vi "AnalogIO.vi"(0 "a_hDevice":i32) -> ()   [LabVIEW 2016]
panel:
  in  "SetAnalogOut":bool
  in  "GetAnalogIn":bool
  in  "GetOnboardAI":bool
  out "AI0":dbl format="%3.2f"
  out "AI7":dbl format="%.2f"
  out "AI6":dbl format="%.2f"
  out "AI3":dbl format="%.2f"
  out "AI2":dbl format="%.2f"
  out "AI1":dbl format="%.2f"
  out "AI4":dbl format="%.2f"
  out "AI5":dbl format="%.2f"
  in  "AO2":dbl format="%.2f"
  in  "AO1":dbl format="%_3f"
  in  "stop":bool
  # "Analog I/O"
  # "Analog Output"
  # "pin 17 (AO1)"
  # "pin 26 (AO2)"
  # "Analog Inptput"
  # "pin 9 (AI1)"
  # "pin 18 (AI2)"
  # "Onboard Analog Input"
  # "thermistor X11"
  # "1V2"
  # "5VIO"
  # "5VUSB"
  # "NTC1 X8"
  # "NTC2 X9"
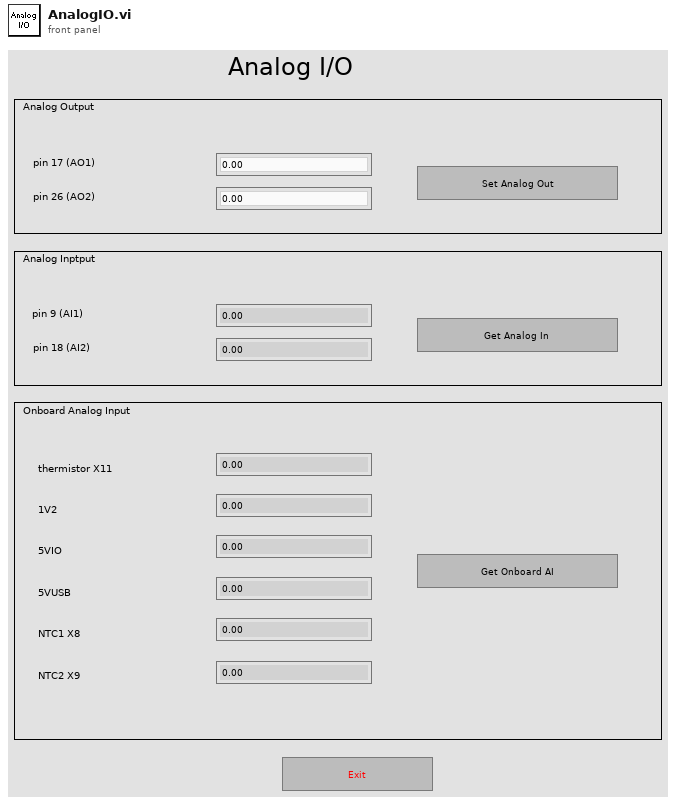
[diagram p1: front panel]
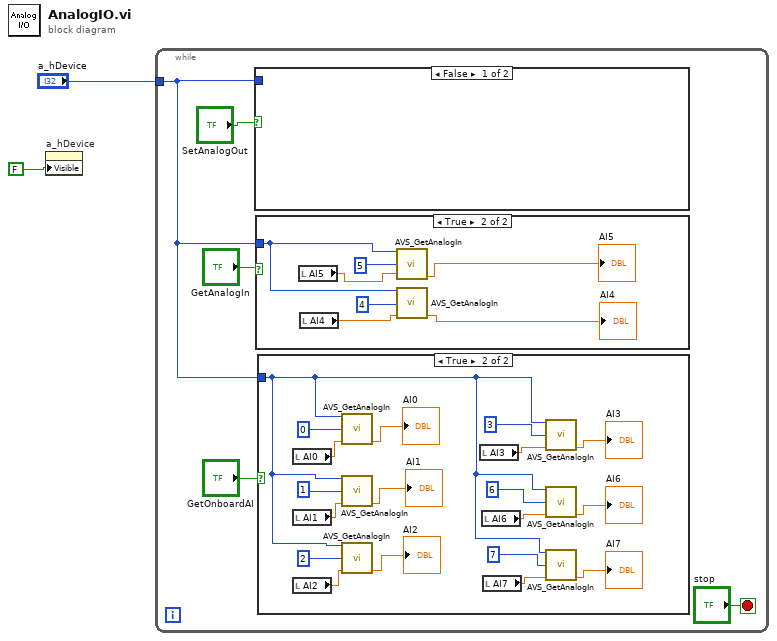
[diagram p0: block diagram]
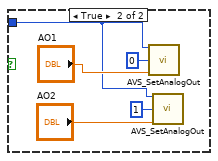
[diagram p4: hidden frame]
diagram:
  n1 = property on="a_hDevice" class="DigNum (strict)"("Visible"=FALSE) -> ()  [unwired: 2 in, 2 out]
  n2 = while {
    tunnel: "a_hDevice" -> [w3]
    stop <- "stop" stop-if-true
    n3 = case shown="False" "SetAnalogOut" {
      tunnel: w3 -> [_ w34]
      frame False {
      }
      frame True {
        n4 = call "AVS_SetAnalogOut.vi"("a_hDevice"=w34, "a_PortId"=u8 0, "a_Value"="AO1") -> ()  [unwired: 12 in, 1 out]
        n5 = call "AVS_SetAnalogOut.vi"("a_hDevice"=w34, "a_PortId"=u8 1, "a_Value"="AO2") -> ()  [unwired: 12 in, 1 out]
      }
    }
    n6 = case shown="True" "GetAnalogIn" {
      tunnel: w3 -> [_ w33]
      frame False {
      }
      frame True {
        n7 = local read "AI5"() -> (w29:dbl)
        n8 = local read "AI4"() -> (w30:dbl)
        n9 = call "AVS_GetAnalogIn.vi"("a_hDevice"=w33, "a_AnalogInId"=u8 5 ("a_PortId"), "a_pAnalogIn"=w29) -> ("a_pAnalogIn"=→"AI5":sgl)  [unwired: 11 in, 1 out]
        n10 = call "AVS_GetAnalogIn.vi"("a_hDevice"=w33, "a_AnalogInId"=u8 4 ("a_PortId"), "a_pAnalogIn"=w30) -> ("a_pAnalogIn"=→"AI4":sgl)  [unwired: 11 in, 1 out]
      }
    }
    n11 = case shown="True" "GetOnboardAI" {
      tunnel: w3 -> [_ w8]
      frame False {
      }
      frame True {
        n12 = local read "AI0"() -> (w17:dbl)
        n13 = local read "AI1"() -> (w18:dbl)
        n14 = local read "AI2"() -> (w19:dbl)
        n15 = call "AVS_GetAnalogIn.vi"("a_hDevice"=w8, "a_AnalogInId"=u8 0 ("a_PortId"), "a_pAnalogIn"=w17) -> ("a_pAnalogIn"=→"AI0":sgl)  [unwired: 11 in, 1 out]
        n16 = call "AVS_GetAnalogIn.vi"("a_hDevice"=w8, "a_AnalogInId"=u8 1 ("a_PortId"), "a_pAnalogIn"=w18) -> ("a_pAnalogIn"=→"AI1":sgl)  [unwired: 11 in, 1 out]
        n17 = call "AVS_GetAnalogIn.vi"("a_hDevice"=w8, "a_AnalogInId"=u8 2 ("a_PortId"), "a_pAnalogIn"=w19) -> ("a_pAnalogIn"=→"AI2":sgl)  [unwired: 11 in, 1 out]
        n18 = local read "AI3"() -> (w12:dbl)
        n19 = local read "AI6"() -> (w13:dbl)
        n20 = local read "AI7"() -> (w14:dbl)
        n21 = call "AVS_GetAnalogIn.vi"("a_hDevice"=w8, "a_AnalogInId"=u8 3 ("a_PortId"), "a_pAnalogIn"=w12) -> ("a_pAnalogIn"=→"AI3":sgl)  [unwired: 11 in, 1 out]
        n22 = call "AVS_GetAnalogIn.vi"("a_hDevice"=w8, "a_AnalogInId"=u8 6 ("a_PortId"), "a_pAnalogIn"=w13) -> ("a_pAnalogIn"=→"AI6":sgl)  [unwired: 11 in, 1 out]
        n23 = call "AVS_GetAnalogIn.vi"("a_hDevice"=w8, "a_AnalogInId"=u8 7 ("a_PortId"), "a_pAnalogIn"=w14) -> ("a_pAnalogIn"=→"AI7":sgl)  [unwired: 11 in, 1 out]
      }
    }
  }
